vi "FTW-ERR-CallChain.vi"(1 "Levels to exclude (1=This VI's caller)":i32=1) -> (0 "Call Chain":string)   [LabVIEW 2013]
panel:
  # "Inputs"
  # "Outputs"
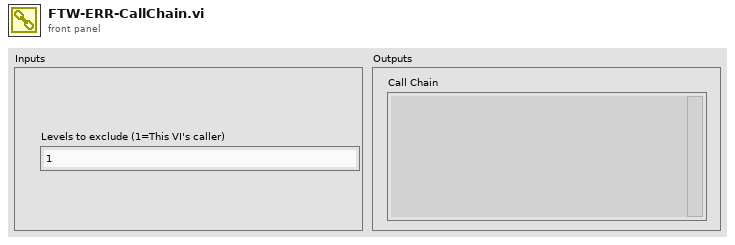
[diagram p1: front panel]
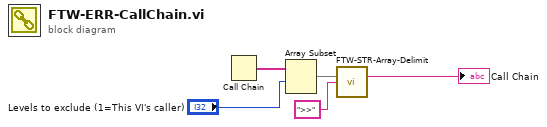
[diagram p0: block diagram]
diagram:
  n1 = Call Chain() -> (call chain=w5:string[])
  n2 = Array Subset(array=w5, index="Levels to exclude (1=This VI's caller)") -> (w3:string[])  [unwired: 1 in]
  n3 = call "FTW-STR-Array-Delimit.vi"("Array of Strings"=w3, "Delimiter"=">>") -> ("Delimited String"=→"Call Chain":string)  [unwired: 13 in]
